vi "Format Graph.vi"(0 "GraphData":T1[](array[typedef])) -> (1 "Dynamic Data Type 2":dynamicdata(waveform), 2 "Dynamic Data Type":dynamicdata(waveform), 3 "Dynamic Data Type 9":dynamicdata(waveform), 4 "Dynamic Data Type 10":dynamicdata(waveform), 6 "Dynamic Data Type 3":dynamicdata(waveform), 8 "Dynamic Data Type 8":dynamicdata(waveform), 10 "Dynamic Data Type 7":dynamicdata(waveform), 12 "Dynamic Data Type 4":dynamicdata(waveform), 13 "Dynamic Data Type 5":dynamicdata(waveform), 14 "Dynamic Data Type 6":dynamicdata(waveform))   [LabVIEW 2012]
uses:
  Nufi/Newfi LDN/subVI/logData.ctl
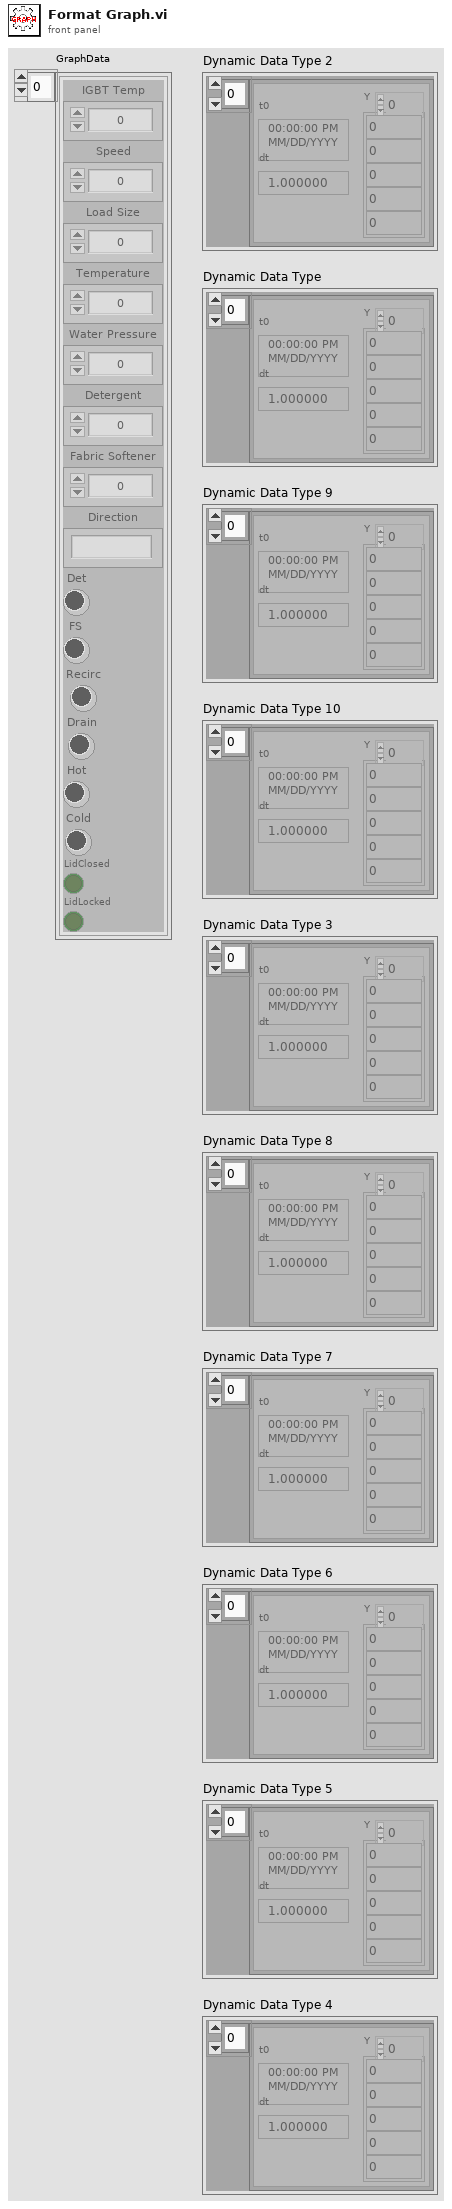
[diagram p1: front panel]
types:
  T1 = typedef "logData.ctl" = cluster{"IGBT Temp":u8, "Speed":u32, "Load Size":u32, "Temperature":u8, "Water Pressure":u32, "Detergent":u32, "Fabric Softener":u32, "Direction":string, "Det":bool, "FS":bool, "Recirc":bool, "Drain":bool, "Hot":bool, "Cold":bool, "LidClosed":bool, "LidLocked":bool}
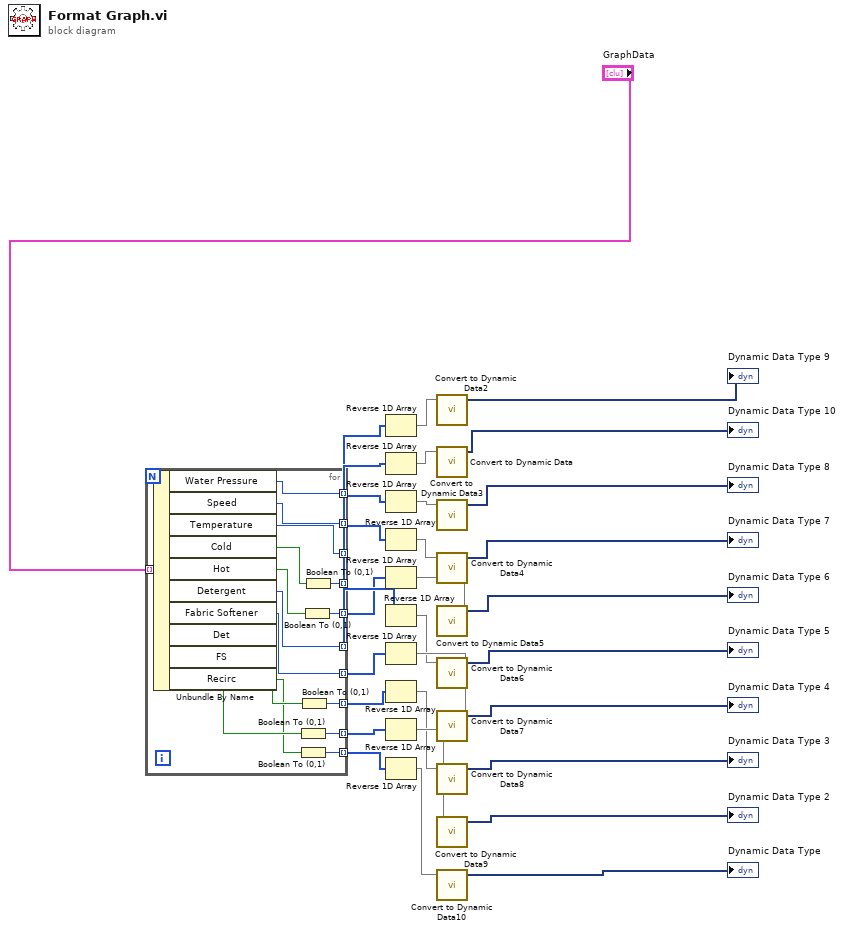
[diagram p0: block diagram]
diagram:
  n1 = for {
    tunnel: "GraphData" -> [w47] mode=indexing
    tunnel: [w46] -> w1 mode=indexing
    tunnel: [w45] -> w2 mode=indexing
    tunnel: [w44] -> w3 mode=indexing
    tunnel: [w43] -> w4 mode=indexing
    tunnel: [w41] -> w5 mode=indexing
    tunnel: [w39] -> w6 mode=indexing
    tunnel: [w38] -> w7 mode=indexing
    tunnel: [w35] -> w8 mode=indexing
    tunnel: [w34] -> w9 mode=indexing
    tunnel: [w32] -> w29 mode=indexing
    n2 = Unbundle By Name(w47) -> ("Water Pressure"=w46:u32, "Speed"=w45:u32, "Temperature"=w44:u8, "Cold"=w42:bool, "Hot"=w40:bool, "Detergent"=w39:u32, "Fabric Softener"=w38:u32, "Det"=w37:bool, "FS"=w36:bool, "Recirc"=w33:bool)
    n3 = Boolean To (0,1)(Boolean=w36) -> (0, 1=w34:i16)
    n4 = Boolean To (0,1)(Boolean=w33) -> (0, 1=w32:i16)
    n5 = Boolean To (0,1)(Boolean=w37) -> (0, 1=w35:i16)
    n6 = Boolean To (0,1)(Boolean=w40) -> (0, 1=w41:i16)
    n7 = Boolean To (0,1)(Boolean=w42) -> (0, 1=w43:i16)
  }
  n8 = Reverse 1D Array(array=w1) -> (reversed array=w13:u32[])
  n9 = Reverse 1D Array(array=w2) -> (reversed array=w11:u32[])
  n10 = Reverse 1D Array(array=w3) -> (reversed array=w15:u8[])
  n11 = Reverse 1D Array(array=w4) -> (reversed array=w17:i16[])
  n12 = Reverse 1D Array(array=w5) -> (reversed array=w19:i16[])
  n13 = Reverse 1D Array(array=w6) -> (reversed array=w21:u32[])
  n14 = Reverse 1D Array(array=w7) -> (reversed array=w23:u32[])
  n15 = Reverse 1D Array(array=w8) -> (reversed array=w25:i16[])
  n16 = Reverse 1D Array(array=w9) -> (reversed array=w27:i16[])
  n17 = Reverse 1D Array(array=w29) -> (reversed array=w30:i16[])
  n18 = call "Convert to Dynamic Data2"("Array"=w13) -> ("Dynamic Data Type"=→"Dynamic Data Type 9":dynamicdata)  [unwired: 3 in]
  n19 = call "Convert to Dynamic Data"("Array"=w11) -> ("Dynamic Data Type"=→"Dynamic Data Type 10":dynamicdata)  [unwired: 3 in]
  n20 = call "Convert to Dynamic Data3"("Array"=w15) -> ("Dynamic Data Type"=→"Dynamic Data Type 8":dynamicdata)  [unwired: 3 in]
  n21 = call "Convert to Dynamic Data4"("Array"=w17) -> ("Dynamic Data Type"=→"Dynamic Data Type 7":dynamicdata)  [unwired: 3 in]
  n22 = call "Convert to Dynamic Data5"("Array"=w19) -> ("Dynamic Data Type"=→"Dynamic Data Type 6":dynamicdata)  [unwired: 3 in]
  n23 = call "Convert to Dynamic Data6"("Array"=w21) -> ("Dynamic Data Type"=→"Dynamic Data Type 5":dynamicdata)  [unwired: 3 in]
  n24 = call "Convert to Dynamic Data7"("Array"=w23) -> ("Dynamic Data Type"=→"Dynamic Data Type 4":dynamicdata)  [unwired: 3 in]
  n25 = call "Convert to Dynamic Data8"("Array"=w25) -> ("Dynamic Data Type"=→"Dynamic Data Type 3":dynamicdata)  [unwired: 3 in]
  n26 = call "Convert to Dynamic Data9"("Array"=w27) -> ("Dynamic Data Type"=→"Dynamic Data Type 2":dynamicdata)  [unwired: 3 in]
  n27 = call "Convert to Dynamic Data10"("Array"=w30) -> ("Dynamic Data Type"=→"Dynamic Data Type":dynamicdata)  [unwired: 3 in]
